vi "Rx Buffer remain.vi"() -> ()   [LabVIEW 2018]
uses:
  <vilib>/Utility/sysdir.llb/System Directory Type.ctl
panel:
  out "End":timestamp format="%<%x %.3X>T"
  out "Start":timestamp format="%<%x %.3X>T"
  out "i":i32 caption="count"
  in  "停止":bool
  in  "タブ制御器":enum32{"Settings"}(tab)
  in  "Time Target (s)":dbl=1.0 caption="Time target(s)"
  in  "IQ Rate (S/s)":dbl[](array[numeric])=[200000000.0, 100000000.0] format="%#.3p"
  in  "Number of Samples":u32[](array[numeric])=[128000, 192000, 256000, 512000, 1024000, 2048000, 4096000] format="%.3p"
  in  "host FIFO":u32[](array[numeric])=[1000000, 10000000] format="%#.3p"
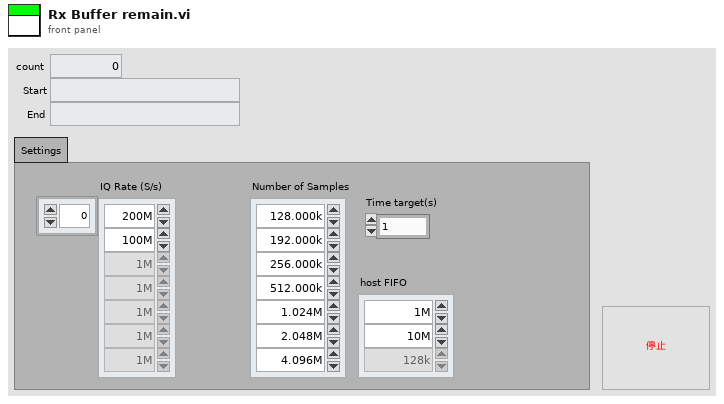
[diagram p1: front panel]
types:
  T1 = typedef "System Directory Type.ctl" = i32
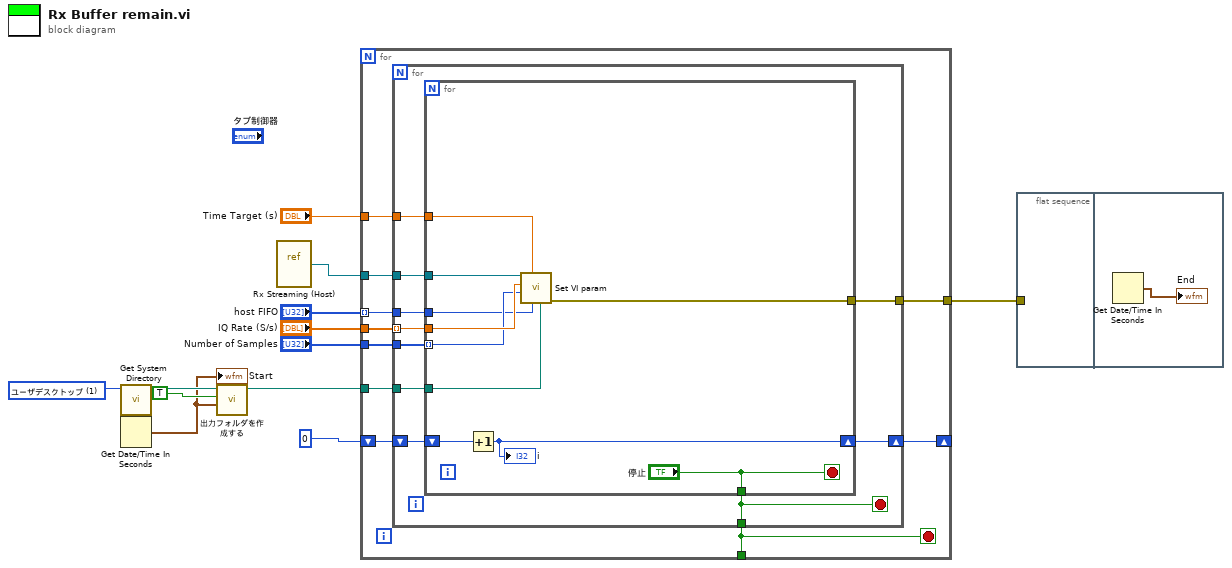
[diagram p0: block diagram]
diagram:
  w8 = T1 1 items=["ユーザホーム"=0, "ユーザデスクトップ"=1, "ユーザドキュメント"=2, "ユーザアプリケーションデータ"=3, "ユーザ設定"=4, "ユーザ一時"=5, "パブリックドキュメント"=6, "パブリックアプリケーションデータ"=7, "パブリック環境設定"=8, "パブリックキャッシュ"=13, "システムコアライブラリ"=9, "システムインストールされたライブラリ"=10, "アプリケーションファイル"=11, "ブート容量ルート"=12] ("system directory type")
  n1 = call <vilib>:"Get System Directory.vi"("system directory type"=w8) -> ("system directory"=w9:path)  [unwired: 10 in]
  n2 = Get Date/Time In Seconds() -> (seconds since 1Jan1904=w7:timestamp)
  "Start" <- w7
  n3 = call "出力フォルダを作成する.vi"("時刻"=w7, "現在時刻のサブフォルダを作成する?(F)"=TRUE, "ルートフォルダ"=w9) -> ("作成されたパス"=w2:path)  [unwired: 5 in, 3 out]
  n4 = vi-ref "Rx Streaming (Host).vi"() -> (w6:refnum<vi>)
  n5 = for {
    tunnel: [w22] -> _
    tunnel: [w18] -> w12
    shift-right: [w20] -> _
    shift-left: 0 -> [w21]
    tunnel: w6 -> [w19]
    tunnel: "host FIFO" -> [w17] mode=indexing
    tunnel: "IQ Rate (S/s)" -> [w16]
    tunnel: "Number of Samples" -> [w15]
    tunnel: w2 -> [w14]
    tunnel: "Time Target (s)" -> [w13]
    stop <- w22 stop-if-true
    n6 = for {
      tunnel: [w28] -> w22
      tunnel: w19 -> [w30]
      tunnel: [w29] -> w18
      shift-right: [w31] -> w20
      shift-left: w21 -> [w32]
      tunnel: w17 -> [w27]
      tunnel: w16 -> [w26] mode=indexing
      tunnel: w15 -> [w25]
      tunnel: w14 -> [w24]
      tunnel: w13 -> [w23]
      stop <- w28 stop-if-true
      n7 = for {
        tunnel: ["停止"] -> w28
        tunnel: w30 -> [w40]
        tunnel: [w34] -> w29
        shift-right: [w41] -> w31
        shift-left: w32 -> [w42]
        tunnel: w27 -> [w37]
        tunnel: w26 -> [w39]
        tunnel: w25 -> [w38] mode=indexing
        tunnel: w24 -> [w36]
        tunnel: w23 -> [w33]
        stop <- "停止" stop-if-true
        n8 = Increment(x=w42) -> (x+1=w41:i32)
        "i" <- w41
        n9 = call "Set VI param.vi"("log path"=w36, "host FIFO depth"=w37, "Time Target (s)"=w33, "number of samples"=w38, "sample rate"=w39, "VI refnum"=w40) -> ("Error Out"=w34:errorcluster)  [unwired: 4 in, 1 out]
      }
    }
  }
  n10 = flat-sequence {
    tunnel: w12 -> [_]
    frame #0 {
    }
    frame #1 {
      n11 = Get Date/Time In Seconds() -> (seconds since 1Jan1904=→"End":timestamp)
    }
  }
